vi "Status String to Cluster.vi"(10 "Status String":string) -> (2 "Status":T1)   [LabVIEW 2019, in "Instrument.Oxford1820.lvclass"]
uses:
  Instrument.Oxford1820.lvclass
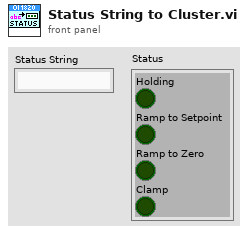
[diagram p1: front panel]
types:
  T1 = cluster{"Holding":bool, "Ramp to Setpoint":bool, "Ramp to Zero":bool, "Clamp":bool}
  T2 = cluster{"[0]":bool, "[1]":bool, "[2]":bool, "[3]":bool}
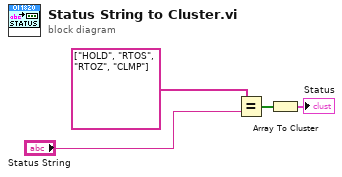
[diagram p0: block diagram]
diagram:
  n1 = Equal?(x=string[] ["HOLD", "RTOS", "RTOZ", "CLMP"] ("Array"), y="Status String") -> (x = y?=w2:bool[])
  n2 = Array To Cluster(array=w2) -> (cluster=→"Status":T2)
